vi "GetImage.vi"(8 "error in (no error)":errorcluster, 10 "inBufferNumber":u32, 11 "Image Acquisition in":refnum<class "Camera.lvclass">) -> (0 "error out":errorcluster, 1 "Cluster":cluster{"processedFPS":dbl, "Buffer Number":u32}, 2 "Image Reference":u16[][](array[numeric]), 3 "Image Acquisition out":refnum<class "Camera.lvclass">)   [LabVIEW 2020, in "Camera.lvclass"]
uses:
  Camera.lvclass
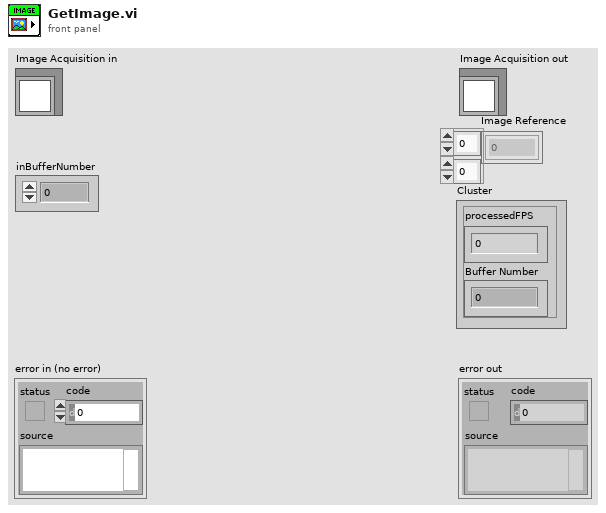
[diagram p1: front panel]
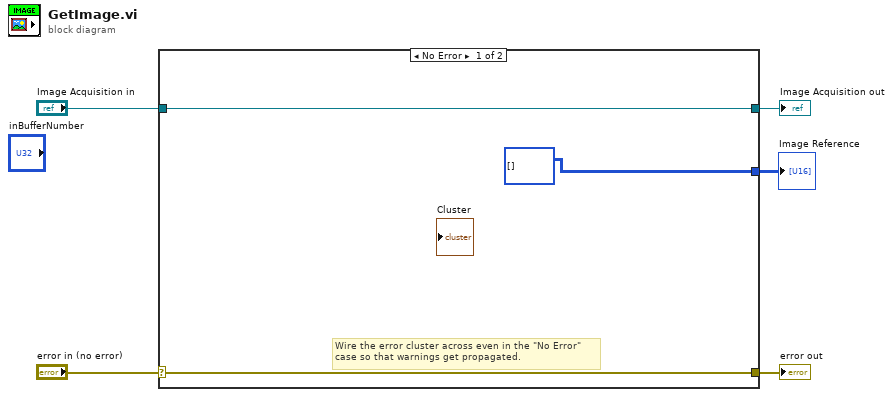
[diagram p0: block diagram]
diagram:
  n1 = case shown="No Error" "error in (no error)" {
    selector: "error in (no error)" -> [w7 w10]
    tunnel: [w7 w10] -> w4
    tunnel: [w8 w9] -> w2
    tunnel: "Image Acquisition in" -> [w8 w9]
    tunnel: [u16[][] [] ("Image Reference") _] -> w1
    frame No Error {
      # "Wire the error cluster across even in the \"No Error\"\ncase so that warnings get propagated."
    }
    frame Error {
    }
  }
  "error out" <- w4
  "Image Acquisition out" <- w2
  "Image Reference" <- w1
